vi "Traffic Light Controller (configurable).vi"(4 "green":bool, 7 "peds stopped":T1) -> (0 "traffic light":T2, 3 "cars stopped":T1)   [LabVIEW 2023]
uses:
  <extravilib>/ChannelInstances/One Element Stream-u16/)Channel.ctl
  <extravilib>/ChannelInstances/One Element Stream-bool/)Channel.ctl
  cd2a572b-c6c3-2d4f-93be-4b20b2e53f24.vi
  04fc8c90-0391-3c46-9268-aa9e1964be30.vi
  <extravilib>/ChannelInstances/One Element Stream-u16/Write With Abort.vi
  <extravilib>/ChannelInstances/One Element Stream-bool/Write With Abort.vi
  <extravilib>/ChannelInstances/One Element Stream-bool/Read With Abort.vi
  <extravilib>/ChannelInstances/One Element Stream-u16/Endpoint.vi
  <extravilib>/ChannelInstances/One Element Stream-bool/Endpoint.vi
  <extravilib>/ChannelInstances/One Element Stream-bool/EndpointRead.vi
  <extravilib>/ChannelInstances/One Element Stream-bool.lvlib
  <extravilib>/ChannelInstances/One Element Stream-u16.lvlib
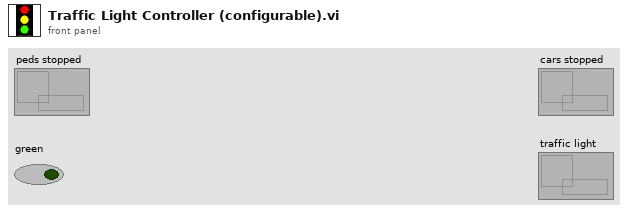
[diagram p1: front panel]
types:
  T1 = typedef "One Element Stream-bool.lvlib/)Channel.ctl" = refnum<queue>
  T2 = typedef "One Element Stream-u16.lvlib/)Channel.ctl" = refnum<queue>
  T3 = enum16{"_Quit_", "Red", "Green", "Yellow", "Config"}
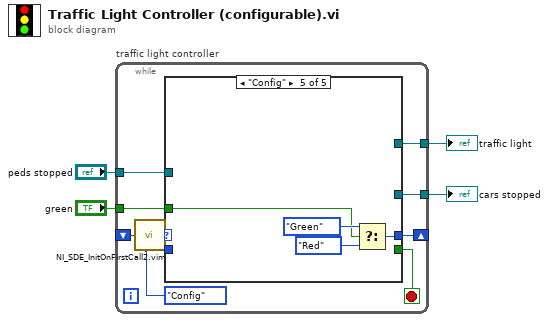
[diagram p0: block diagram]
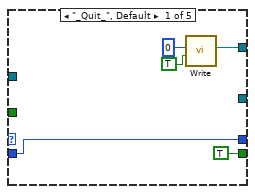
[diagram p2: hidden frame]
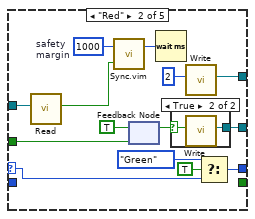
[diagram p3: hidden frame]
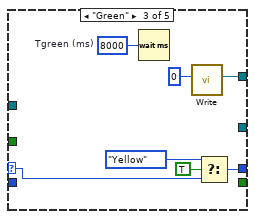
[diagram p5: hidden frame]
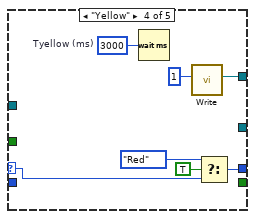
[diagram p6: hidden frame]
diagram:
  n1 = while "traffic light controller" {
    tunnel: "peds stopped" -> [w12]
    tunnel: [w11] -> w4
    tunnel: [w10] -> w3
    tunnel: "green" -> [w9]
    shift-right: [w7] -> _
    shift-left: _ -> [w6]
    stop <- w13 stop-if-true
    w8 = T3."Config"
    n2 = call "NI_SDE_InitOnFirstCall2.vim"("input"=w6, "master enum"=w8) -> ("output enum"=w5:T3)  [unwired: 1 in]
    n3 = case shown="\"Config\"" w5 {
      selector: w5 -> [_ w32 w41 w48 _]
      tunnel: [TRUE _ _ _ _] -> w13
      tunnel: [w14 w31 w40 w47 w51] -> w7
      tunnel: w12 -> [_ w29 _ _ _]
      tunnel: [w16 w27 w35 w45 _] -> w11
      tunnel: [_ w26 _ _ _] -> w10
      tunnel: w9 -> [_ w19 _ _ w49]
      tunnel: w8 -> [w14 _ _ _ _]
      frame "_Quit_", Default {
        n4 = call <extravilib>:"Write.vi"("last element? (F)"=TRUE, "element"=u16 0) -> ("channel"=w16:T2)  [unwired: 8 in, 1 out]
      }
      frame "Red" {
        w23 = u32 1000  # safety margin
        n5 = call <extravilib>:"Read.vi"("channel"=w29) -> ("element"=w24:bool)  [unwired: 7 in, 3 out]
        n6 = call "Sync.vim"("a"=w23, "b"=w24) -> ("a'"=w22:u32)  [unwired: 24 in, 1 out]
        n7 = feedback-in #1(TRUE) -> ()
        n8 = feedback #1(w19) -> (w20:bool)
        n9 = Wait (ms)(milliseconds to wait=w22) -> ()  [unwired: 1 out]
        n10 = case shown="True" w20 {
          selector: w20 -> [_ w33]
          tunnel: [_ w34] -> w26
          frame False {
          }
          frame True {
            n11 = call <extravilib>:"Write.vi"("element"=w33) -> ("channel"=w34:T1)  [unwired: 9 in, 1 out]
          }
        }
        n12 = call <extravilib>:"Write.vi"("element"=u16 2) -> ("channel"=w27:T2)  [unwired: 9 in, 1 out]
        n13 = Select(t=T3."Green", s=TRUE, f=w32) -> (s? t:f=w31:T3)
      }
      frame "Green" {
        w38 = u32 8000  # Tgreen (ms)
        n14 = Wait (ms)(milliseconds to wait=w38) -> ()  [unwired: 1 out]
        n15 = call <extravilib>:"Write.vi"("element"=u16 0) -> ("channel"=w35:T2)  [unwired: 9 in, 1 out]
        n16 = Select(t=T3."Yellow", s=TRUE, f=w41) -> (s? t:f=w40:T3)
      }
      frame "Yellow" {
        w42 = u32 3000  # Tyellow (ms)
        n17 = Wait (ms)(milliseconds to wait=w42) -> ()  [unwired: 1 out]
        n18 = call <extravilib>:"Write.vi"("element"=u16 1) -> ("channel"=w45:T2)  [unwired: 9 in, 1 out]
        n19 = Select(t=T3."Red", s=TRUE, f=w48) -> (s? t:f=w47:T3)
      }
      frame "Config" {
        n20 = Select(t=T3."Green", s=w49, f=T3."Red") -> (s? t:f=w51:T3)
      }
    }
  }
  "traffic light" <- w4
  "cars stopped" <- w3
